vi "MapAndWrite.vi"(4 "error in (no error)":errorcluster, 5 "String_Cast_of_Info":string, 6 "Commands":T1=enum."Delete mission", 7 "NetworkStreamWriter in":refnum<class "NetworkStreamWriter.lvclass">) -> (0 "error out":errorcluster, 3 "NetworkStreamWriter out":refnum<class "NetworkStreamWriter.lvclass">)   [LabVIEW 2013]
doc: "It takes in an enum identifying what type of OCU command it is as well as a string cast of the infomation to send and writes it to the NetworkStream for Main.vi to recieve. The information needs to be in the correct or the forebrain will break wile parsing it or creat jibberish. Refer to Forebrain/Sense/GetOCUCommands.vi to determine the appropriate format.\n\nWritten by: Victoria Coleman 04/14"
uses:
  NetworkStreamWriter.lvclass
  OCU/CommandMessages.ctl
  ToRIO.ctl
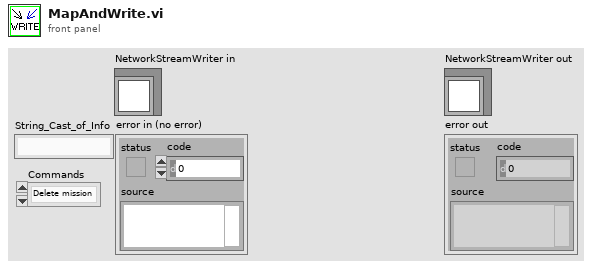
[diagram p1: front panel]
types:
  T1 = typedef "CommandMessages.ctl" = enum16{"Pass", "OverrideMode", "Add mission", "Delete mission", "Change constants"}
  T2 = typedef "ToRIO.ctl" = cluster{"Commands":T1, "Variant":variant}
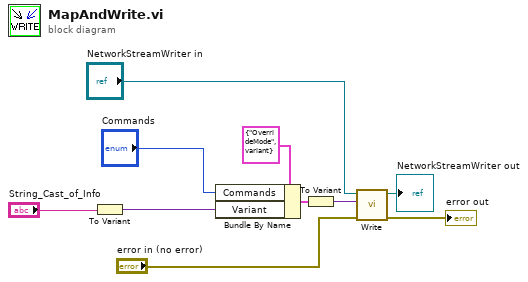
[diagram p0: block diagram]
diagram:
  n1 = To Variant(anything="String_Cast_of_Info") -> (Variant=w2:variant)
  n2 = Bundle By Name(cluster=T2 {"Commands"=enum."OverrideMode", "Variant"=variant} ("To RIO"), "Commands"="Commands", "Variant"=w2) -> (w10:T2)
  n3 = To Variant(anything=w10) -> (Variant=w9:variant)
  n4 = call "Write.vi"("error in (no error)"="error in (no error)", "element"=w9, "NetworkStreamWriter in"="NetworkStreamWriter in") -> ("error out"=→"error out":errorcluster, "NetworkStreamWriter out"=→"NetworkStreamWriter out":refnum<class "NetworkStreamWriter.lvclass">)  [unwired: 7 in]
